vi "trim tabs.vi"(1 "string":string) -> (0 "result string":string)   [LabVIEW 2018]
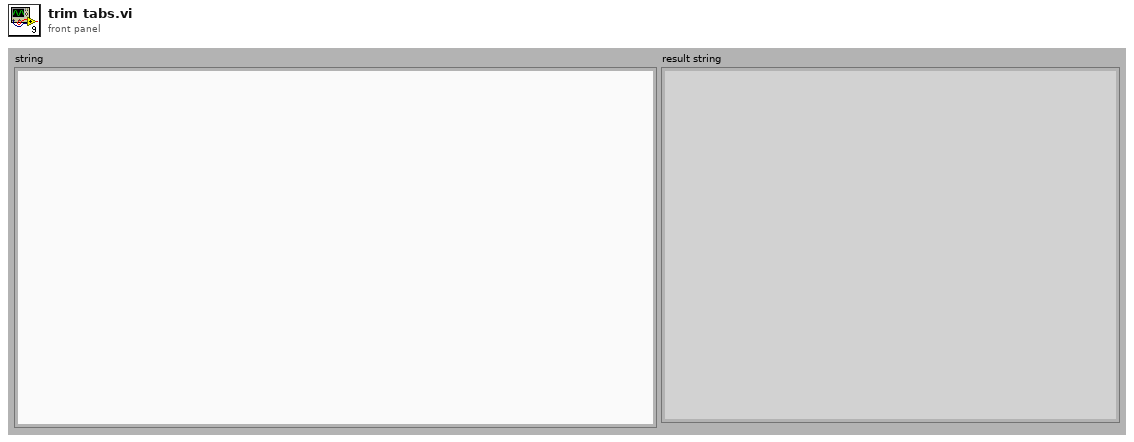
[diagram p1: front panel]
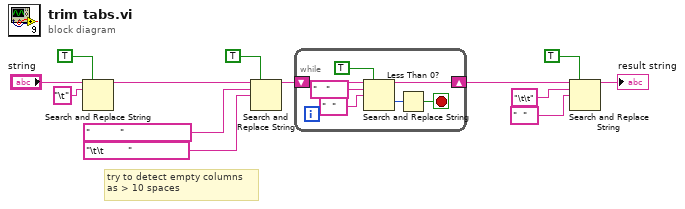
[diagram p0: block diagram]
diagram:
  # "try to detect empty columns\nas > 10 spaces"
  n1 = Search and Replace String(replace all?=TRUE ("replace all? (F)"), input string="string", search string="\t") -> (result string=w1:string)  [unwired: 5 in, 3 out]
  n2 = Search and Replace String(replace all?=TRUE ("replace all? (F)"), input string=w1, search string="          ", replace string="\t\t        " ("search string")) -> (result string=w2:string)  [unwired: 4 in, 3 out]
  n3 = while {
    shift-right: [w16] -> w3
    shift-left: w2 -> [w20]
    stop <- w14 stop-if-true
    n4 = Search and Replace String(replace all?=TRUE ("replace all? (F)"), input string=w20, search string="   ", replace string="  " ("search string")) -> (result string=w16:string, offset past replacement=w15:i32)  [unwired: 4 in, 2 out]
    n5 = Less Than 0?(x=w15) -> (x < 0?=w14:bool)
  }
  n6 = Search and Replace String(replace all?=TRUE ("replace all? (F)"), input string=w3, search string="\t\t", replace string="  " ("search string")) -> (result string=→"result string":string)  [unwired: 4 in, 3 out]
